vi "Fetch Waveform Measurement In Memory.vi"(6 "Measurement Number (0: Measurement 1)":i32(ring) items=["Measurement 1", "Measurement 2", "Measurement 3", "Measurement 4"], 7 "Destination Channel (1: Channel 2)":u16(ring)=1 items=["Channel 1", "Channel 2", "Channel 3", "Channel 4", "Math", "D0", "D1", "D2", "D3", "D4", "D5", "D6", "D7", "D8", "D9", "D10", "D11", "D12", "D13", "D14", "D15", "Reference 1", "Reference 2", "Reference 3", "Reference 4", "Amplitude", "Frequency", "Phase"], 8 "error in (no error)":errorcluster, 9 "Measurement Function (21: Period)":i32(ring)=21 items=["Amplitude", "Area", "Burst Width", "Cycle Area", "Voltage Mean (cycle)", "Voltage RMS (cycle)", "Delay", "Fall Time", "Frequency", "Voltage High", "Voltage Low", "Voltage Max", "Voltage Mean", "Voltage Min", "Negative Duty Cycle", "Negative Edges Count", "Negative Overshoot", "Negative Pulses Count", "Negative Pulse Width", "Positive Duty Cycle", "Positive Edges Count", "Period", "Phase", "Vpp", "Positive Overshoot", "Positive Pulses Count", "Positive Pulse Width", "Rise Time", "Voltage RMS", "Total Overshoot", "Histogram Hits", "Histogram Median", "Histogram Peak Hits", "Histogram Sigma 1", "Histogram Sigma 2", "Histogram Sigma 3", "Standard Deviation", "Waveform Count"], 10 "Channel (0: Channel 1)":u16(ring) items=["Channel 1", "Channel 2", "Channel 3", "Channel 4", "Math", "D0", "D1", "D2", "D3", "D4", "D5", "D6", "D7", "D8", "D9", "D10", "D11", "D12", "D13", "D14", "D15", "Reference 1", "Reference 2", "Reference 3", "Reference 4", "Amplitude", "Frequency", "Phase"], 11 "VISA resource name":refnum<visa-resource-name>) -> (0 "error out":errorcluster, 2 "Measurement Value":dbl, 3 "VISA resource name out":refnum<visa-resource-name>)   [LabVIEW 2016, in "Tektronix DPO MSO 2000 4000 Series.lvlib"]
doc: "This VI fetches the displayed measurement value which is specified by the <B>Measurement Number</B>. \n\nFirstly, initiates an acquisition on the channel that you specify in the <B>Channel</B> control. After the acquisition completes, the Fetch Displayed Waveform Measurement VI performs displayed waveform measurement on the channel you specify and returns a measurement value. You can specify a measurement type, such as rise time, frequency, and voltage peak-to-peak, with this VI. Use the Fetch Displayed Waveform Measurement VI separately for any other waveform measurement on a channel without initiating another acquisition.\n\n<B>Notes:</B>\n\nThe <B>Fetch Waveform Measurement</B> VI returns the immediate measurement (which is what is typically done) while this VI returns the specified displayed measurement."
uses:
  Tektronix DPO MSO 2000 4000 Series.lvlib
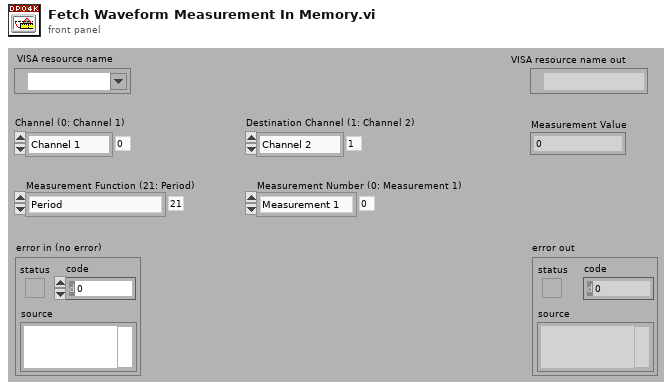
[diagram p1: front panel]
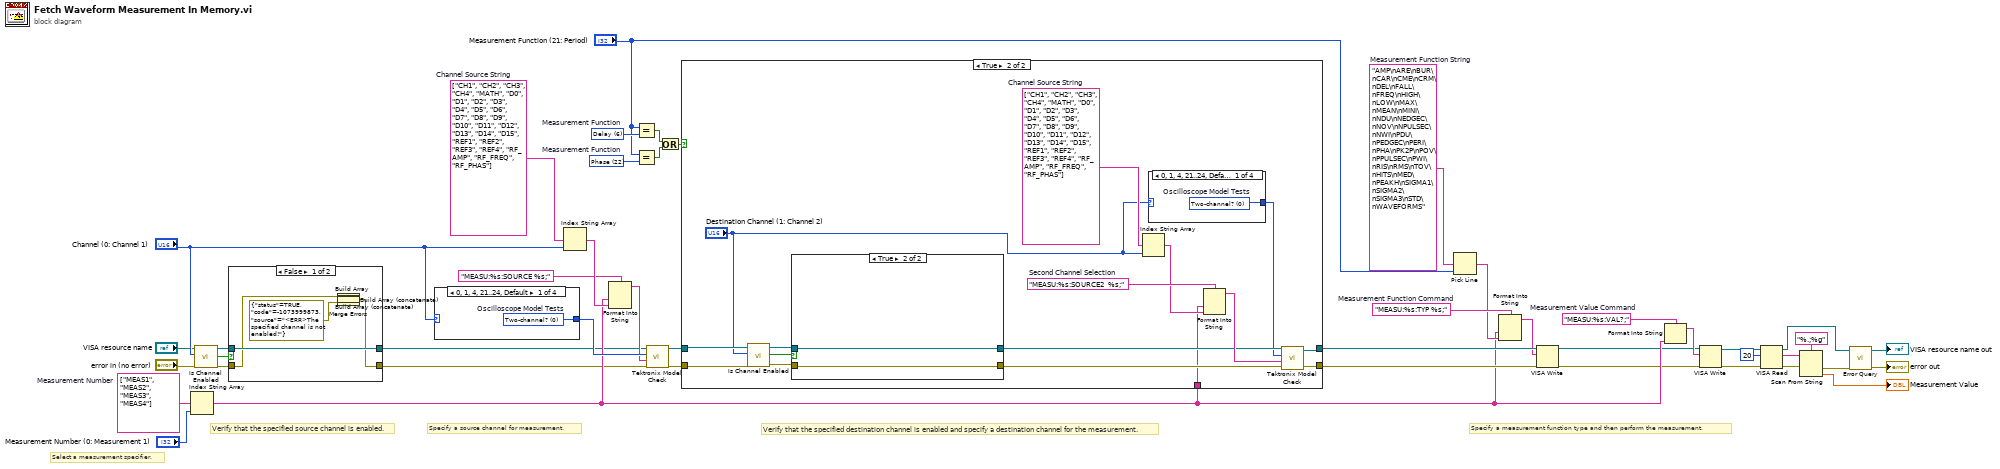
[diagram p0: block diagram]
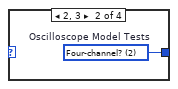
[diagram p3: hidden frame]
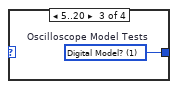
[diagram p4: hidden frame]
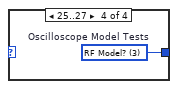
[diagram p5: hidden frame]
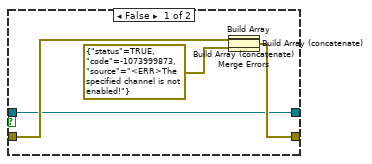
[diagram p6: hidden frame]
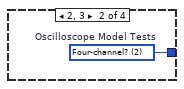
[diagram p7: hidden frame]
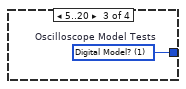
[diagram p8: hidden frame]
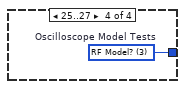
[diagram p9: hidden frame]
diagram:
  w11 = string[] ["MEAS1", "MEAS2", "MEAS3", "MEAS4"]  # Measurement Number
  w13 = "MEASU:%s:VAL?;"  # Measurement Value Command
  w28 = 22 items=["Amplitude", "Area", "Burst Width", "Cycle Area", "Voltage Mean (cycle)", "Voltage RMS (cycle)", "Delay", "Fall Time", "Frequency", "Voltage High", "Voltage Low", "Voltage Max", "Voltage Mean", "Voltage Min", "Negative Duty Cycle", "Negative Edges Count", "Negative Overshoot", "Negative Pulses Count", "Negative Pulse Width", "Positive Duty Cycle", "Positive Edges Count", "Period", "Phase", "Vpp", "Positive Overshoot", "Positive Pulses Count", "Positive Pulse Width", "Rise Time", "Voltage RMS"]  # Measurement Function
  w29 = 6 items=["Amplitude", "Area", "Burst Width", "Cycle Area", "Voltage Mean (cycle)", "Voltage RMS (cycle)", "Delay", "Fall Time", "Frequency", "Voltage High", "Voltage Low", "Voltage Max", "Voltage Mean", "Voltage Min", "Negative Duty Cycle", "Negative Edges Count", "Negative Overshoot", "Negative Pulses Count", "Negative Pulse Width", "Positive Duty Cycle", "Positive Edges Count", "Period", "Phase", "Vpp", "Positive Overshoot", "Positive Pulses Count", "Positive Pulse Width", "Rise Time", "Voltage RMS"]  # Measurement Function
  w37 = string[] ["CH1", "CH2", "CH3", "CH4", "MATH", "D0", "D1", "D2", "D3", "D4", "D5", "D6", "D7", "D8", "D9", "D10", "D11", "D12", "D13", "D14", "D15", "REF1", "REF2", "REF3", "REF4", "RF_AMP", "RF_FREQ", "RF_PHAS"]  # Channel Source String
  w44 = "MEASU:%s:TYP %s;"  # Measurement Function Command
  w45 = "AMP\nARE\nBUR\nCAR\nCME\nCRM\nDEL\nFALL\nFREQ\nHIGH\nLOW\nMAX\nMEAN\nMINI\nNDU\nNEDGEC\nNOV\nNPULSEC\nNWI\nPDU\nPEDGEC\nPERI\nPHA\nPK2P\nPOV\nPPULSEC\nPWI\nRIS\nRMS\nTOV\nHITS\nMED\nPEAKH\nSIGMA1\nSIGMA2\nSIGMA3\nSTD\nWAVEFORMS"  # Measurement Function String
  # "Select a measurement specifier."
  # "Specify a measurement function type and then perform the measurement."
  # "Specify a source channel for measurement."
  # "Verify that the specified destination channel is enabled and specify a destination channel for the measurement."
  # "Verify that the specified source channel is enabled."
  n1 = Index String Array(1:"Measurement Number (0: Measurement 1)", 2:w11) -> (0:w9:string)  [unwired: 1 in]
  n2 = call "Is Channel Enabled.vi"("error in (no error)"="error in (no error)", "Channel (0: Channel 1)"="Channel (0: Channel 1)", "VISA resource name"="VISA resource name") -> ("error out"=w40:errorcluster, "Enabled"=w41:bool, "VISA resource name out"=w39:refnum<visa-resource-name>)  [unwired: 6 in]
  n3 = case shown="False" w41 {
    tunnel: w40 -> [w50 w53]
    tunnel: w39 -> [w51 w54]
    tunnel: [w51 w54] -> w4
    tunnel: [w49 w53] -> w3
    frame False {
      n4 = Build Array(w50, errorcluster {"status"=TRUE, "code"=-1073999873, "source"="<ERR>The specified channel is not enabled!"} ("error out")) -> (w48:errorcluster[])
      n5 = Build Array (concatenate)(w48) -> (w47:errorcluster[])
      n6 = Build Array (concatenate)(w47) -> (w46:errorcluster[])
      n7 = Merge Errors(w46) -> (w49:errorcluster)
    }
    frame True {
    }
  }
  n8 = case shown="0, 1, 4, 21..24, Default" "Channel (0: Channel 1)" {
    tunnel: [w55 w56 w57 w58] -> w38
    frame 0, 1, 4, 21..24, Default {
      w55 = u16 0 items=["Two-channel?", "Digital Model?", "Four-channel?", "RF Model?"]  # Oscilloscope Model Tests
    }
    frame 2, 3 {
      w56 = u16 2 items=["Two-channel?", "Digital Model?", "Four-channel?", "RF Model?"]  # Oscilloscope Model Tests
    }
    frame 5..20 {
      w57 = u16 1 items=["Two-channel?", "Digital Model?", "Four-channel?", "RF Model?"]  # Oscilloscope Model Tests
    }
    frame 25..27 {
      w58 = u16 3 items=["Two-channel?", "Digital Model?", "Four-channel?", "RF Model?"]  # Oscilloscope Model Tests
    }
  }
  n9 = Index String Array(1:"Channel (0: Channel 1)", 2:w37) -> (0:w35:string)  [unwired: 1 in]
  n10 = Format Into String(format string="MEASU:%s:SOURCE %s;", w9, w35) -> (resulting string=w33:string)  [unwired: 2 in, 1 out]
  n11 = Equal?(x="Measurement Function (21: Period)", y=w29) -> (x = y?=w30:bool)
  n12 = Equal?(x="Measurement Function (21: Period)", y=w28) -> (x = y?=w31:bool)
  n13 = call "Tektronix Model Check.vi"("error in (no error)"=w3, "Command String"=w33, "Oscilloscope Model Tests (3: RF Model?)"=w38, "VISA resource name"=w4) -> ("error out"=w7:errorcluster, "VISA resource name out"=w8:refnum<visa-resource-name>)  [unwired: 6 in]
  n14 = Or(x=w30, y=w31) -> (x .or. y?=w27:bool)
  n15 = case shown="True" w27 {
    tunnel: w8 -> [w60 w69]
    tunnel: w7 -> [w59 w68]
    tunnel: [w60 w67] -> w25
    tunnel: [w59 w66] -> w24
    tunnel: w9 -> [_ w63]
    frame False {
    }
    frame True {
      w73 = string[] ["CH1", "CH2", "CH3", "CH4", "MATH", "D0", "D1", "D2", "D3", "D4", "D5", "D6", "D7", "D8", "D9", "D10", "D11", "D12", "D13", "D14", "D15", "REF1", "REF2", "REF3", "REF4", "RF_AMP", "RF_FREQ", "RF_PHAS"]  # Channel Source String
      w65 = "MEASU:%s:SOURCE2  %s;"  # Second Channel Selection
      n16 = call "Is Channel Enabled.vi"("error in (no error)"=w68, "Channel (0: Channel 1)"="Destination Channel (1: Channel 2)", "VISA resource name"=w69) -> ("error out"=w72:errorcluster, "Enabled"=w70:bool, "VISA resource name out"=w71:refnum<visa-resource-name>)  [unwired: 6 in]
      n17 = case shown="True" w70 {
        tunnel: w71 -> [w84 w89]
        tunnel: w72 -> [w86 w88]
        tunnel: [w84 w89] -> w74
        tunnel: [w85 w88] -> w75
        frame False {
          n18 = Build Array(w86, errorcluster {"status"=TRUE, "code"=-1073999873, "source"="<ERR>The specified channel is not enabled!"} ("error out")) -> (w83:errorcluster[])
          n19 = Build Array (concatenate)(w83) -> (w82:errorcluster[])
          n20 = Build Array (concatenate)(w82) -> (w81:errorcluster[])
          n21 = Merge Errors(w81) -> (w85:errorcluster)
        }
        frame True {
        }
      }
      n22 = Index String Array(1:"Destination Channel (1: Channel 2)", 2:w73) -> (0:w64:string)  [unwired: 1 in]
      n23 = case shown="0, 1, 4, 21..24, Default" "Destination Channel (1: Channel 2)" {
        tunnel: [w77 w78 w79 w80] -> w61
        frame 0, 1, 4, 21..24, Default {
          w77 = u16 0 items=["Two-channel?", "Digital Model?", "Four-channel?", "RF Model?"]  # Oscilloscope Model Tests
        }
        frame 2, 3 {
          w78 = u16 2 items=["Two-channel?", "Digital Model?", "Four-channel?", "RF Model?"]  # Oscilloscope Model Tests
        }
        frame 5..20 {
          w79 = u16 1 items=["Two-channel?", "Digital Model?", "Four-channel?", "RF Model?"]  # Oscilloscope Model Tests
        }
        frame 25..27 {
          w80 = u16 3 items=["Two-channel?", "Digital Model?", "Four-channel?", "RF Model?"]  # Oscilloscope Model Tests
        }
      }
      n24 = Format Into String(format string=w65, w63, w64) -> (resulting string=w76:string)  [unwired: 2 in, 1 out]
      n25 = call "Tektronix Model Check.vi"("error in (no error)"=w75, "Command String"=w76, "Oscilloscope Model Tests (3: RF Model?)"=w61, "VISA resource name"=w74) -> ("error out"=w66:errorcluster, "VISA resource name out"=w67:refnum<visa-resource-name>)  [unwired: 6 in]
    }
  }
  n26 = Pick Line(multi-line string=w45, line index="Measurement Function (21: Period)") -> (output string=w32:string)  [unwired: 1 in]
  n27 = Format Into String(format string=w44, w9, w32) -> (resulting string=w23:string)  [unwired: 2 in, 1 out]
  n28 = VISA Write(VISA resource name=w25, write buffer=w23, error in (no error)=w24) -> (VISA resource name out=w6:refnum<visa-resource-name>, error out=w5:errorcluster)  [unwired: 1 out]
  n29 = Format Into String(format string=w13, w9) -> (resulting string=w12:string)  [unwired: 2 in, 1 out]
  n30 = VISA Write(VISA resource name=w6, write buffer=w12, error in (no error)=w5) -> (VISA resource name out=w21:refnum<visa-resource-name>, error out=w20:errorcluster)  [unwired: 1 out]
  n31 = VISA Read(VISA resource name=w21, byte count=u32 20, error in (no error)=w20) -> (VISA resource name out=w17:refnum<visa-resource-name>, read buffer=w16:string, error out=w18:errorcluster)  [unwired: 1 out]
  n32 = Scan From String(format string="%.;%g", input string=w16, error in=w18) -> (error out=w15:errorcluster, output 1=→"Measurement Value":dbl)  [unwired: 2 in, 2 out]
  n33 = call "Error Query.vi"("error in (no error)"=w15, "VISA resource name"=w17) -> ("error out"=→"error out":errorcluster, "VISA resource name out"=→"VISA resource name out":refnum<visa-resource-name>)  [unwired: 6 in, 2 out]
